vi "Dashboard Main.vi"() -> ()   [LabVIEW 2014]
uses:
  <vilib>/event_ctls.llb/eventvkey.ctl
  <vilib>/Rock Robotics/WPI/Dashboard/WPI_DashboardLogging Global.vi
  <vilib>/Rock Robotics/Network Tables/SD Read Boolean Array.vi
  <vilib>/Rock Robotics/Network Tables/SD Read Number.vi
  <vilib>/Utility/config.llb/Write Key (String).vi
  <vilib>/Utility/config.llb/Write Key (I32).vi
  <vilib>/Utility/config.llb/NI_LVConfig.lvlib
panel:
  in  "TCP":refnum<k5>
  out "Camera IP":string
  out "Image Message":string="Timeout in Camera Communications"
  in  "Dashboard Tab":T1(tab)
  out "Right Joystick Shift":bool
  out "Left Joystick Shift":bool
  out "Right Joystick Arcade":bool
  out "Left Joystick Arcade":bool
  out "Right Joystick X":dbl
  out "Left Joystick Y":dbl
  out "Left Joystick X":dbl
  out "Right Joystick Y":dbl
  out "Intake Open/Close":dbl
  out "Tote Motor Signal":dbl
  out "Tote Elevator Signal":dbl
  out "Top Limit Switch":bool
  out "Bottom Limit Switch":bool
  out "Tote Elevator Pot":dbl
  out "Accelerometer":dbl
  out "Gyro Angle":dbl
  out "Motor Signal":dbl
  out "Encoder":dbl
  out "BR Feedback":dbl
  out "FR Feedback":dbl
  out "BL Feedback":dbl
  out "FL Feedback":dbl
  out "BR Signal":dbl
  out "FR Signal":dbl
  out "BL Signal":dbl
  out "FL Signal":dbl
  in  "Camera Settings":T2={"Frame Rate"=30, "Compression"=30, "Size"=1} {"Frame Rate" scale=1.0..30.0; "Size" items=["640x480", "320x240", "160x120"]}
  out "MotorChart R":cluster{"Numeric":dbl, "Numeric":dbl}(graph)
  out "MotorChart L":T3(graph)
  out "MotorSliders R":cluster{"MotorSlide1":dbl, "MotorSlide2":dbl} {"MotorSlide2" scale=-1.0..1.0 scale format="%#_2e"; "MotorSlide1" scale=-1.0..1.0 scale format="%#_2e"}
  out "MotorSliders L":T4 {"MotorSlide4 2" scale=0.0..14.0 scale format="%#_2e"; "MotorSlide2" scale=-1.0..1.0 scale format="%#_2e"; "MotorSlide1" scale=-1.0..1.0 scale format="%#_2e"}
  out "Gyro":dbl(knob) scale=0.0..360.0
  out "JS1 Z":dbl(slide) scale=-1.0..1.0 scale format="%#_2e"
  out "JS1 Graph":cluster{"X":dbl, "Y":dbl}[](graph)
  out "JS1 Buttons":T5
  out "JS2 Z":dbl(slide) scale=-1.0..1.0 scale format="%#_2e"
  out "JS2 Graph":cluster{"X":dbl, "Y":dbl}[](graph)
  out "JS2 Buttons":T5
  out "Mode":T6(ring)=enum."Auto Disabled"
  in  "DB Camera Config":bool
  out "fps":dbl format="%#.1g"
  out "Mbps":dbl format="%#.1g"
  out "Mbps 2":bool
  out "Camera Image":T7(plugin-control)
  in  "Vision":u16(ring) items=["Camera Off", "USB Camera SW", "USB Camera HW", "IP Camera"]
  in  "Rec Mode":enum32{"Stop", "Record", "Playback"}(radio)
  in  "DB/String 9":string
  in  "DB/String 8":string
  in  "DB/String 7":string
  in  "DB/String 6":string
  in  "DB/String 5":string
  in  "DB/String 4":string
  in  "DB/String 3":string
  in  "DB/String 2":string
  in  "DB/String 1":string
  in  "DB/String 0":string
  in  "DB/Slider 0":dbl(slide) scale=0.0..5.0
  in  "DB/Slider 1":dbl(slide) scale=0.0..5.0
  in  "DB/Slider 2":dbl(slide) scale=0.0..5.0
  in  "DB/Slider 3":dbl(slide) scale=0.0..5.0
  out "DB/LED 3":bool
  out "DB/LED 2":bool
  out "DB/LED 1":bool
  out "DB/LED 0":bool
  in  "DB/Button 3":bool
  in  "DB/Button 2":bool
  in  "DB/Button 1":bool
  in  "DB/Button 0":bool caption="New Name"
  in  "Test Slider":dbl(slide) scale=0.0..100.0 scale format="%#_3g"
  in  "On/Off":bool caption="Solenoid"
  in  "Test Name":u16(ring) items=["Select the test to run...", "Example Test", "-------------------------------", "List of tests is built in robot code.", "Replace with your own automated tests."]
  in  "Test Tree":string(tree)
  in  "Motor":cluster{"Value":dbl, "Enable":bool} {"Value" scale=-1.0..1.0 scale format="%#_3g"}
  out "Progress":T8 {"Test Progress" scale=0.0..100.0}
  in  "Rev/Fwd":cluster{"Forward":bool, "Reverse":bool}
  in  "Test Ring":u16(ring) items=["Monochrome", "Color"]
  in  "Listbox":i32(listbox)
  out "Tree":string(tree)
  out "Boolean":bool
  # "Drivetrain Values"
  # "Other Sensors"
  # "Drivetrain Values"
  # "Craaa"
  # "Tote Elevator"
  # "Tote Intake"
  # "Left"
  # "Front"
  # "Right"
  # "Battery"
  # "This tab is a great place for autonomous settings and robot-specific values.\nPlace controls and indicators inside this tab and match name to\nDashboard Variables on robot. You can also delete this comment."
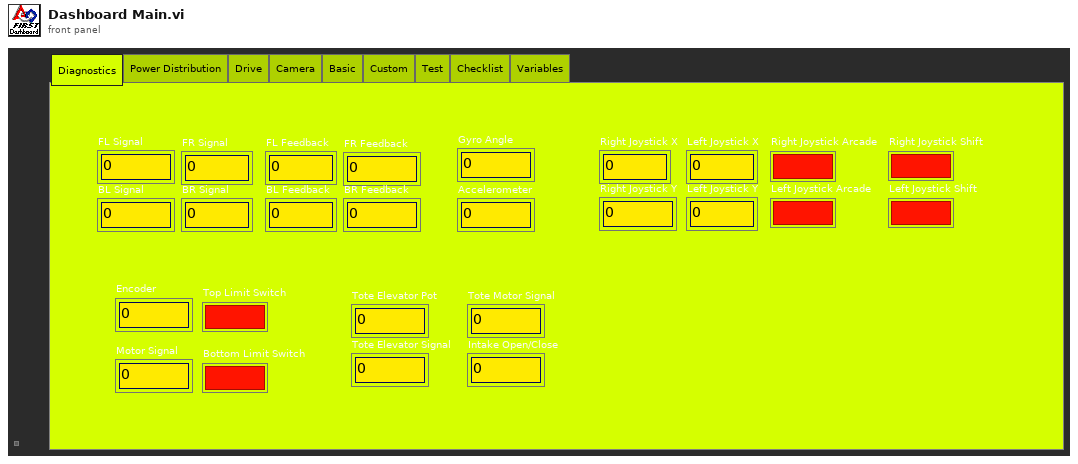
[diagram p1: front panel]
types:
  T1 = enum32{"Diagnostics", "Power Distribution", "Drive", "Camera", "Basic", "Custom", "Test", "Checklist", "Variables"}
  T2 = cluster{"Frame Rate":i32, "Compression":i32, "Size":u16}
  T3 = cluster{"Numeric":dbl, "Numeric":dbl, "Battery V":dbl}
  T4 = cluster{"MotorSlide1":dbl, "MotorSlide2":dbl, "MotorSlide4 2":dbl}
  T5 = cluster{bool, bool, bool, bool, bool, bool, bool, bool, bool, bool, bool, bool}
  T6 = enum8{"Tele-Op Disabled", "Tele-Op Enabled", "Auto Disabled", "Auto Enabled", "Test Disabled", "Test Enabled", "Disconnected", "No Code", "E-Stop"}
  T7 = typedef "IMAQ Image.ctl" = refnum<image>
  T8 = cluster{"Test Progress":u8, "Test Progress Text":string}
  T9 = enum32{"Drive", "Basic", "Custom", "Test", "Checklist", "Variables"}
  T10 = typedef "Image Type" = u32
  T11 = cluster{"Camera Image":refnum<vi>, "Dashboard Tab":refnum<vi>, "Boolean":refnum<vi>, "Vision":refnum<vi>, "Rec Mode":refnum<vi>, "Test Slider":refnum<vi>, "On/Off ":refnum<vi>, "Test Ring":refnum<vi>, "Rev/Fwd":refnum<vi>, "Test Name":refnum<vi>, "Motor":refnum<vi>, "Progress":refnum<vi>, "CheckList":refnum<vi>, "Tree":refnum<vi>, "Test Tree":refnum<vi>}
  T12 = cluster{"Error Strings":string, "Disable Counts":cluster{u16, u16}, "Rail Faults":cluster{u16, u16, u16}, "Robot IP":string, "DB Mode":u8, "Event Info":cluster{"Name":string, "Type":u8, "Number":u16, "Replay":u8}, "Camera Addr":string}
  T13 = cluster{"Storage":cluster{"Disk Free":u64, "RAM Block":u32, "RAM free":u32}, "CPU Utilization":cluster{"CPU % ISR":sgl, "CPU % Time Crit":sgl, "CPU % Timed Str":sgl, "CPU % High":sgl, "CPU % Above":sgl, "CPU % Normal":sgl, "CPU % Low":sgl}, "CAN":cluster{"% Bus Utilization":sgl, "Bus Off Cnt":u32, "TX_FIFO Full Cnt":u32, "Receive Error Cnt":u8, "Transmit Error Cnt":u8}, "HID":cluster{"HID Outputs":u32, "Rumble Low":u16, "Rumble High":u16}[]}
  T14 = cluster{"Status bits":cluster{"Test Mode":bool, "Autonomous":bool, "Enabled":bool, "Code Start":bool, "Brownout":bool, "Reserved 2":bool, "Reserved 3":bool, "E-Stop":bool}, "Code Trace":cluster{"Disabled":bool, "TeleOp":bool, "Auto":bool, "Test":bool}, "Controller Type":enum16{"unknown", "cRIO", "roboRio"}, "Code?":enum16{"unknown", "noCode", "code"}, "Battery V":dbl}
  T15 = cluster{"Control Bits":cluster{"TestMode":bool, "Autonomous":bool, "Enabled":bool, "FMS Present":bool, bool, bool, bool, "E-Stop":bool}, "Team Station ":u8, "Countdown":sgl, "Joystick Values":cluster{"Axes":dbl[], "Buttons":bool[], "POVs":i16[]}[]}
  T16 = cluster{"Axes":dbl[], "Buttons":bool[], "POVs":i16[]}[]
  T17 = cluster{"Axes":dbl[], "Buttons":bool[], "POVs":i16[]}
  T18 = cluster{"Buttons[0]":bool, "Buttons[1]":bool, "Buttons[2]":bool, "Buttons[3]":bool, "Buttons[4]":bool, "Buttons[5]":bool, "Buttons[6]":bool, "Buttons[7]":bool, "Buttons[8]":bool, "Buttons[9]":bool, "Buttons[10]":bool, "Buttons[11]":bool}
  T19 = cluster{"Boolean Array[0]":bool, "Boolean Array[1]":bool, "Boolean Array[2]":bool, "Boolean Array[3]":bool, "Boolean Array[4]":bool, "Boolean Array[5]":bool, "Boolean Array[6]":bool, "Boolean Array[7]":bool, "Boolean Array[8]":bool}
  T20 = cluster{"Numeric Array[0]":dbl, "Numeric Array[1]":dbl, "Numeric Array[2]":dbl, "Numeric Array[3]":dbl, "Numeric Array[4]":dbl, "Numeric Array[5]":dbl, "Numeric Array[6]":dbl, "Numeric Array[7]":dbl, "Numeric Array[8]":dbl}
  T21 = typedef "NI_LVConfig.lvlib/Config Data RefNum.ctl" = refnum<k1>
  T22 = cluster{"Operation":enum16{"Update", "Clear"}, "Color Box":u32}[]
  T23 = typedef "eventvkey.ctl" = enum16{"ASCII", "Enter", "Return", "Shift", "Ctrl", "Alt", "Cmd", "Opt", "Caps", "NumLock", "Clear", "Break", "Up", "Down", "Left", "Right", "Insert", "Delete", "Home", "End", "PageUp", "PageDown", "Escape", "Help", "Pause", "ScrollLock", "F1", "F2", "F3", "F4", "F5", "F6", "F7", "F8", "F9", "F10", "F11", "F12", "F13", "F14", "F15", "F16", "F17", "F18", "F19", "F20", "F21", "F22", "F23", "F24", "Play", "VolumeUp", "VolumeDown", "Mute", "Two Byte Char"}
  T24 = cluster{"Image Size":bool, "Image Type":bool, "Pixel Value":bool, "ROI Information":bool, "Zoom Factor":bool}
  T25 = enum8{"Enabled", "Disabled", "Disabled and Grayed Out"}
  T26 = cluster{"Operation":enum16{"Update", "Clear"}, "Color Box":u32}
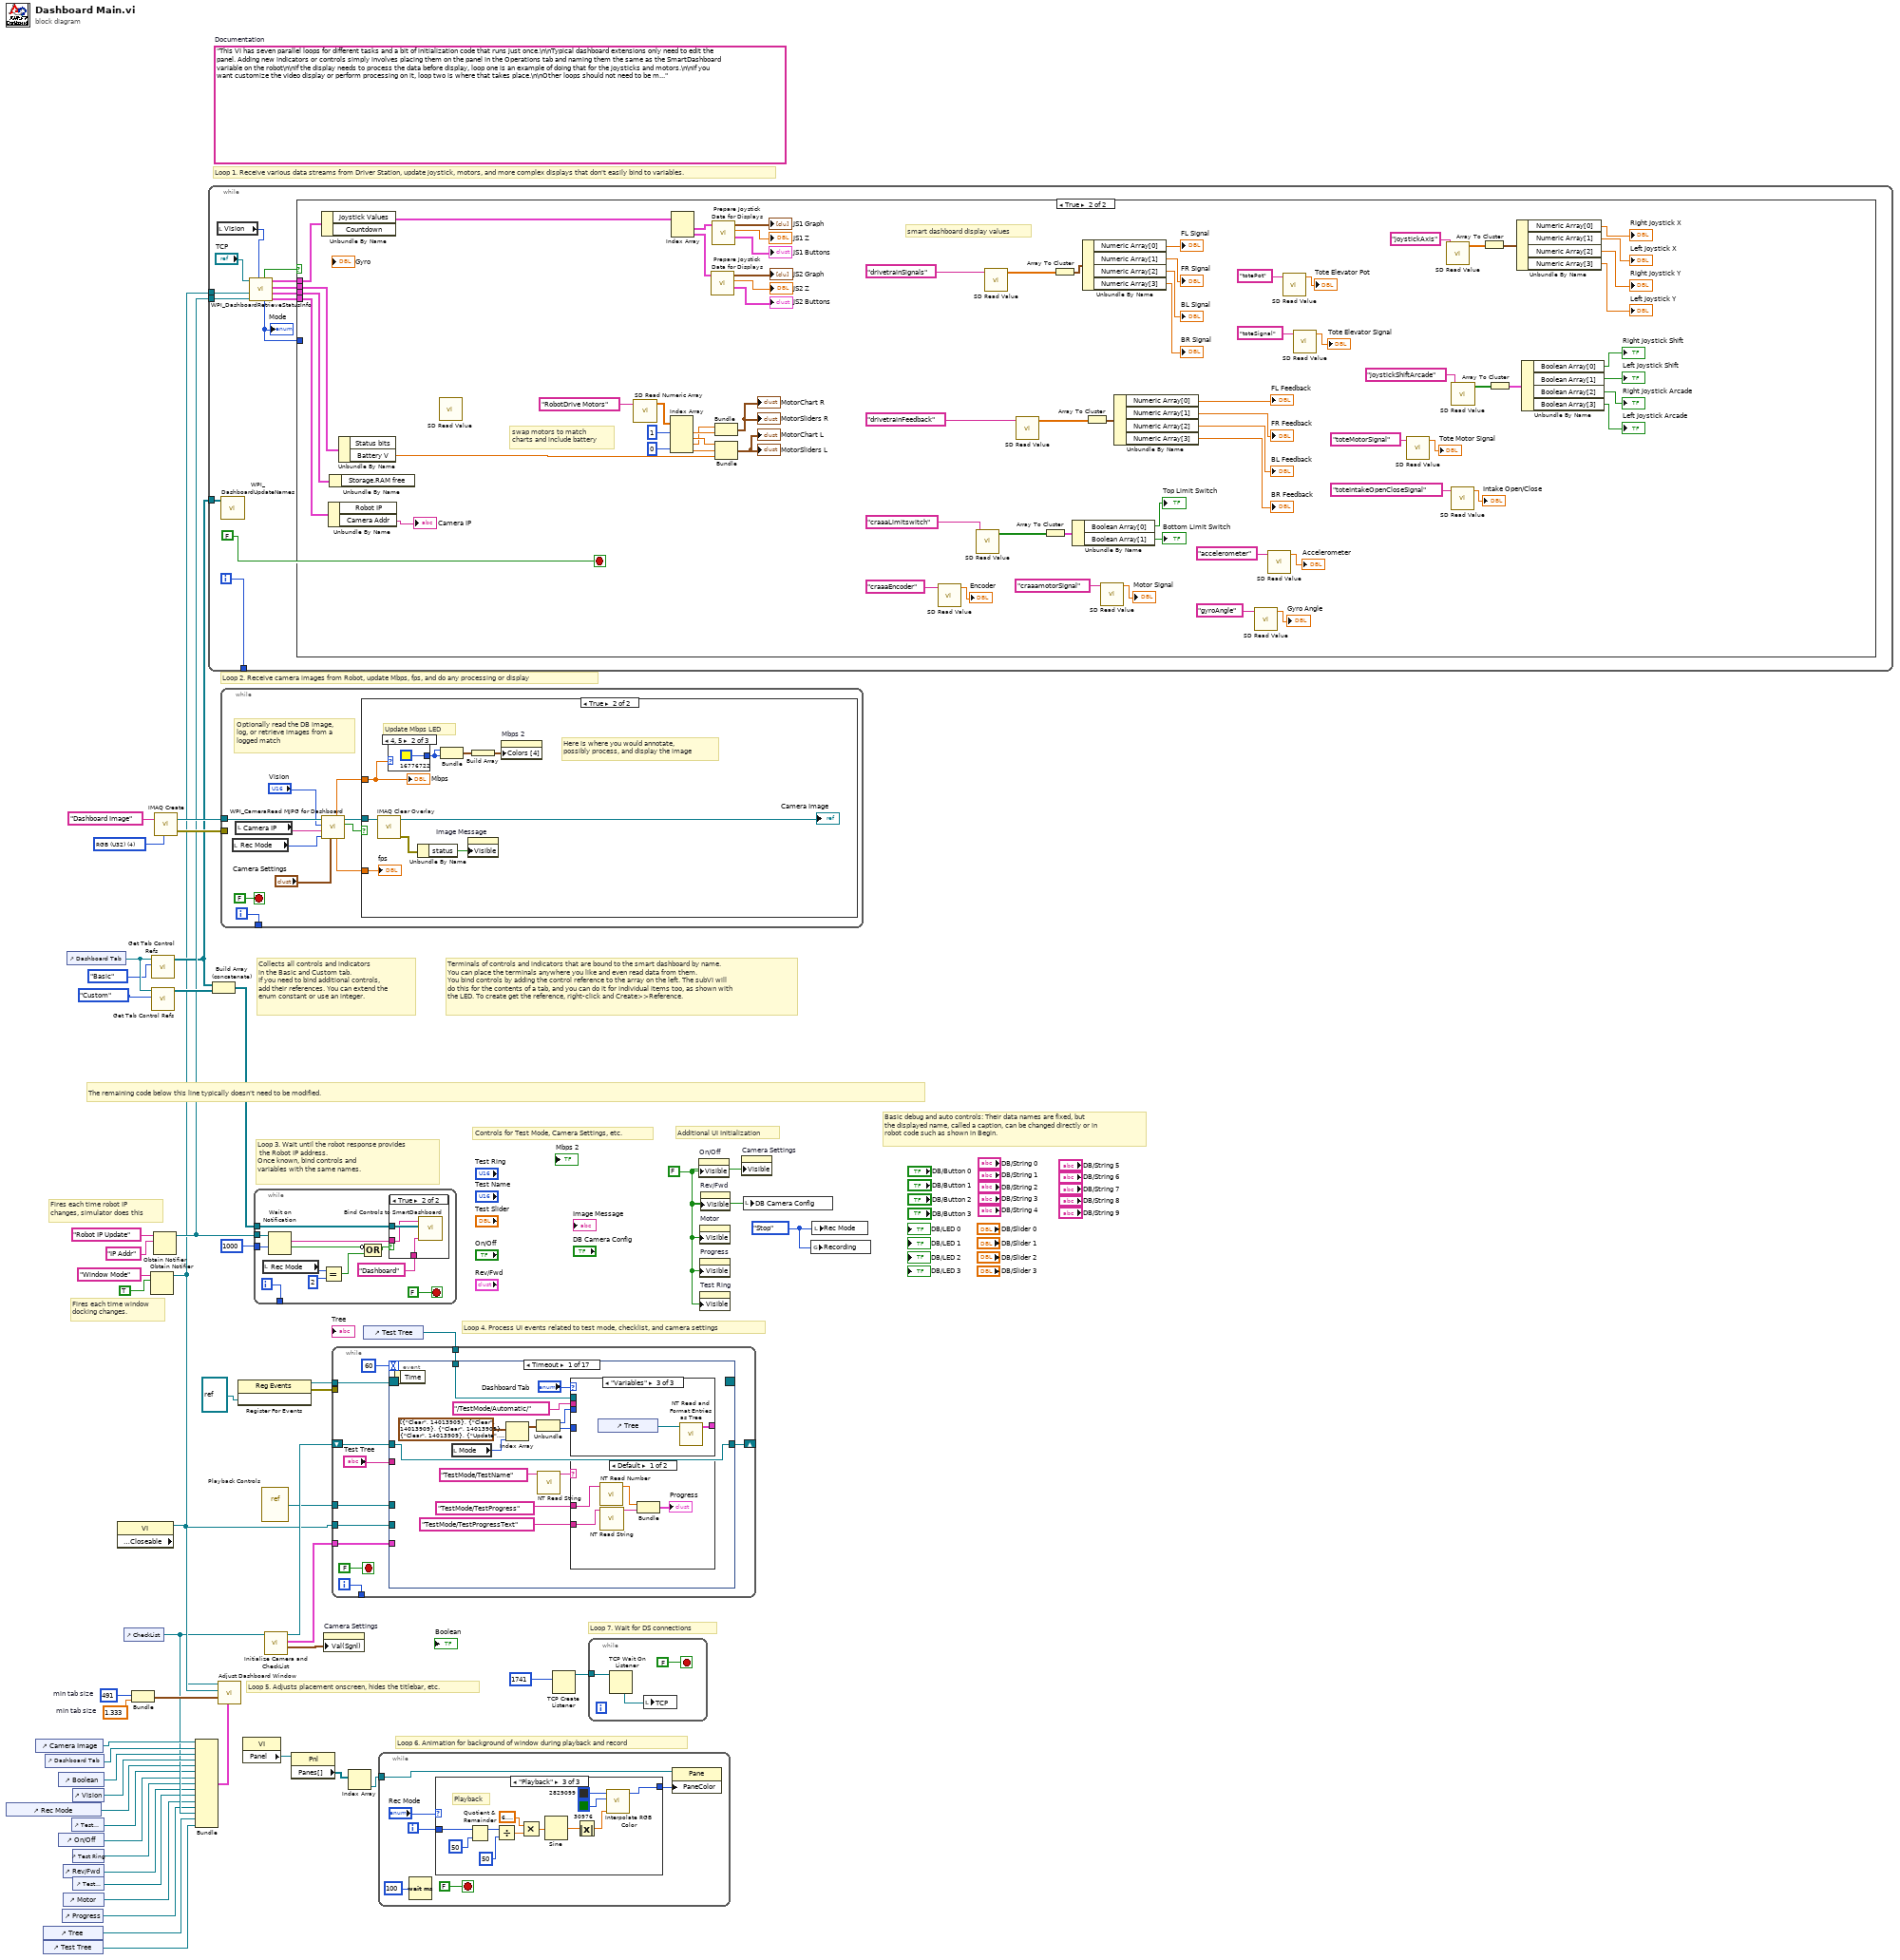
[diagram p0: block diagram]
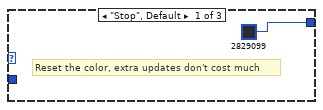
[diagram p3: hidden frame]
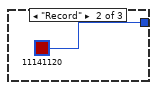
[diagram p4: hidden frame]
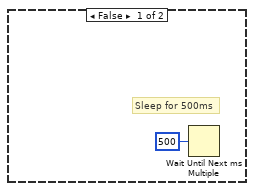
[diagram p6: hidden frame]
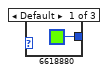
[diagram p7: hidden frame]
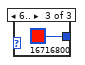
[diagram p8: hidden frame]
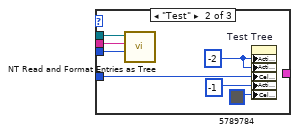
[diagram p10: hidden frame]
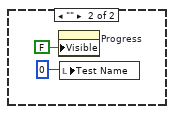
[diagram p11: hidden frame]
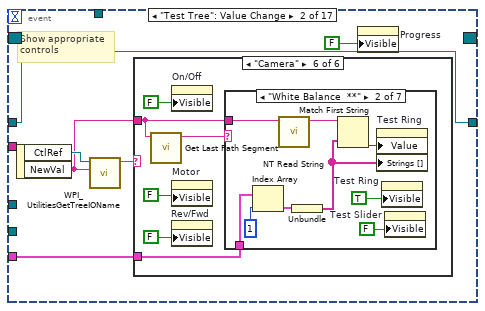
[diagram p12: hidden frame]
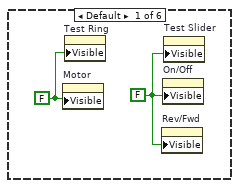
[diagram p13: hidden frame]
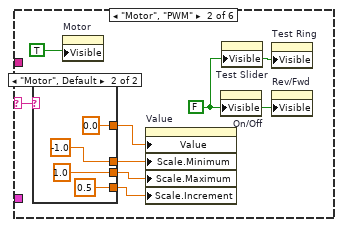
[diagram p14: hidden frame]
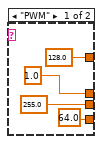
[diagram p15: hidden frame]
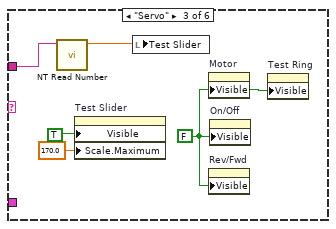
[diagram p16: hidden frame]
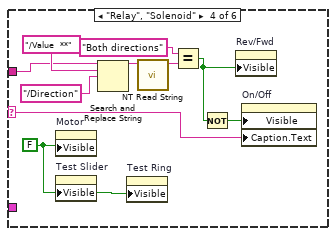
[diagram p17: hidden frame]
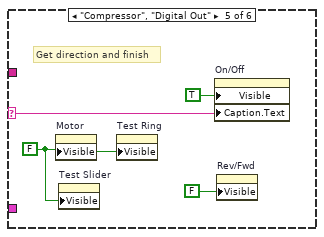
[diagram p18: hidden frame]
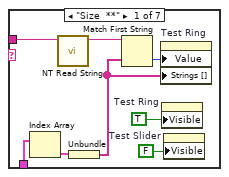
[diagram p19: hidden frame]
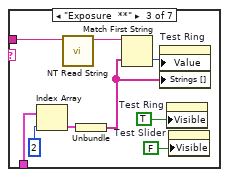
[diagram p20: hidden frame]
diagram:
  w24 = 491  # min tab size
  w23 = 1.333  # min tab size
  w32 = enum32{"Stop", "Record", "Playback"}."Stop" ("Rec Mode")
  w6 = FALSE ("Visible")
  (unwired) "This VI has seven parallel loops for different tasks and a bit of initialization code that runs just once.\n\nTypical dashboard extensions only need to edit the panel. Adding new indicators or controls simply involves placing them on the panel in the Operations tab and naming them the same as the SmartDashboard variable on the robot\n\nIf the display needs to process the data before display, loop one is an example of doing that for the joysticks and motors.\n\nIf you want customize the video display or perform processing on it, loop two is where that takes place.\n\nOther loops should not need to be modified. They are pretty standard, and document the task they perform."  # Documentation
  w52 = T10 4 items=["Grayscale (U8)", "Grayscale (I16)", "Grayscale (SGL)", "Complex (CSG)", "RGB (U32)", "HSL (U32)", "RGB (U64)"] ("Image Type")
  # "Loop 7. Wait for DS connections"
  # "Basic debug and auto controls: Their data names are fixed, but\nthe displayed name, called a caption, can be changed directly or in\nrobot code such as shown in Begin."
  # "Controls for Test Mode, Camera Settings, etc."
  # "Additional UI Initialization"
  # "Loop 6. Animation for background of window during playback and record"
  # "Fires each time robot IP\nchanges, simulator does this"
  # "Fires each time window\ndocking changes."
  # "Collects all controls and indicators\nin the Basic and Custom tab.\nIf you need to bind additional controls,\nadd their references. You can extend the\nenum constant or use an integer."
  # "The remaining code below this line typically doesn't need to be modified."
  # "Loop 4. Process UI events related to test mode, checklist, and camera settings"
  # "Terminals of controls and indicators that are bound to the smart dashboard by name.\nYou can place the terminals anywhere you like and even read data from them.\nYou bind controls by adding the control reference to the array on the left. The subVI will\ndo this for the contents of a tab, and you can do it for individual items too, as shown with\nthe LED. To create get the reference, right-click and Create>>Reference."
  # "Loop 3. Wait until the robot response provides\n the Robot IP address.\nOnce known, bind controls and\nvariables with the same names."
  # "Loop 5. Adjusts placement onscreen, hides the titlebar, etc."
  # "Loop 1. Receive various data streams from Driver Station, update joystick, motors, and more complex displays that don't easily bind to variables."
  # "Loop 2. Receive camera images from Robot, update Mbps, fps, and do any processing or display"
  n1 = control-ref of="Rec Mode"() -> (w12:refnum<vi>)
  n2 = control-ref of="Camera Image"() -> (w27:refnum<vi>)
  n3 = control-ref of="Tree"() -> (w16:refnum<vi>)
  n4 = control-ref of="Test Tree"() -> (w15:refnum<vi>)
  n5 = control-ref of="Dashboard Tab"() -> (w26:refnum<vi>)
  n6 = control-ref of="Boolean"() -> (w21:refnum<vi>)
  n7 = control-ref of="On/Off"() -> (w10:refnum<vi>)
  n8 = control-ref of="Progress"() -> (w7:refnum<vi>)
  n9 = control-ref of="Rev/Fwd"() -> (w8:refnum<vi>)
  n10 = control-ref of="Motor"() -> (w13:refnum<vi>)
  n11 = control-ref of="Dashboard Tab"() -> (w30:refnum<vi>)
  n12 = control-ref of="Test Slider"() -> (w11:refnum<vi>)
  n13 = control-ref of="Vision"() -> (w25:refnum<vi>)
  n14 = control-ref of="Test Ring"() -> (w9:refnum<vi>)
  n15 = control-ref of="Test Name"() -> (w14:refnum<vi>)
  n16 = property class="VI" props=["Front Panel.Closeable"]() -> (reference out=w31:refnum<vi>)  [unwired: 2 in, 2 out]
  n17 = control-ref of="CheckList"() -> (w17:refnum<vi>)
  n18 = Bundle("min tab size"=w24, "min tab size"=w23) -> (w22:cluster{"min tab size":i32, "min tab size":dbl})  [unwired: 1 in]
  n19 = Obtain Notifier(name (unnamed)="Window Mode", notification data type=TRUE) -> (notifier out=w3:refnum<notifier>)  [unwired: 2 in, 2 out]
  n20 = call <vilib>:"Get Tab Control Refs.vi"("Page Index"=T9."Basic" ("Dashboard Tab"), "TabControl in"=w30) -> ("ControlsOnPage"=w4:refnum<vi>[])  [unwired: 9 in]
  n21 = call <vilib>:"Get Tab Control Refs.vi"("Page Index"=T9."Custom" ("Dashboard Tab"), "TabControl in"=w30) -> ("ControlsOnPage"=w29:refnum<vi>[])  [unwired: 9 in]
  n22 = Obtain Notifier(name (unnamed)="Robot IP Update", notification data type="IP Addr" ("name (unnamed)")) -> (notifier out=w5:refnum<notifier>)  [unwired: 2 in, 2 out]
  n23 = call "IMAQ Create"("Image Name"="Dashboard Image", "Image Type"=w52) -> ("New Image"=w50:T7, "error out"=w49:errorcluster)  [unwired: 2 in, 1 out]
  n24 = Bundle("Camera Image"=w27, "Dashboard Tab"=w26, "Boolean"=w21, "Vision"=w25, "Rec Mode"=w12, "Test Slider"=w11, "On/Off"=w10, "Test Ring"=w9, "Rev/Fwd"=w8, "Test Name"=w14, "Motor"=w13, "Progress"=w7, "CheckList"=w17, "Tree"=w16, "Test Tree"=w15) -> (w18:T11)  [unwired: 1 in]
  n25 = while {
    tunnel: [w64] -> _
    tunnel: w5 -> [w58]
    tunnel: w4 -> [w57]
    tunnel: w3 -> [w53]
    i -> [w64]
    stop <- FALSE stop-if-true
    n26 = local read "Vision"() -> (w55:u16)
    n27 = call <vilib>:"WPI_DashboardUpdateNames.vi"("Controls on Tab"=w57) -> ()  [unwired: 11 in]
    n28 = call <vilib>:"WPI_DashboardRetrieveStatusInfo.vi"("Vision"=w55, "Binding Refnum"=w58, "Window Mode Notifier"=w53, "TCP Cnx"="TCP") -> ("Power and Errors"=w59:T12, "Robot Metrics"=w62:T13, "Status Info"=w63:T14, "Control Info"=w60:T15, "Robot Mode"=w56:T6, "Process?"=w61:bool)  [unwired: 2 in]
    "Mode" <- w56
    n29 = case shown="True" w61 {
      tunnel: w63 -> [_ w139]
      tunnel: w62 -> [_ w138]
      tunnel: w60 -> [_ w137]
      tunnel: w59 -> [_ w136]
      tunnel: w56 -> [_ _]
      frame False {
      }
      frame True {
        # "smart dashboard display values"
        # "swap motors to match\ncharts and include battery"
        n30 = Unbundle By Name(w137) -> ("Joystick Values"=w124:T16)  [unwired: 1 out]
        n31 = Unbundle By Name(w136) -> ("Camera Addr"=→"Camera IP":string)  [unwired: 1 out]
        n32 = Unbundle By Name(w138) -> ()  [unwired: 1 out]
        n33 = Unbundle By Name(w139) -> ("Battery V"=w125:dbl)  [unwired: 1 out]
        n34 = call-poly <vilib>:"SD Read Value.vi"() -> ()  [unwired: 9 in, 3 out]
        n35 = call <vilib>:"SD Read Numeric Array.vi"("Name"="RobotDrive Motors") -> ("Numeric Array"=w127:dbl[])  [unwired: 8 in, 2 out]
        n36 = Index Array(array=w127, index #1=1, index #4=0) -> (element #1=w131:dbl, element #2=w132:dbl, element #3=w130:dbl, element #4=w135:dbl)  [unwired: 2 in]
        n37 = Index Array(array=w124) -> (element #1=w123:T17, element #2=w118:T17)  [unwired: 2 in]
        n38 = call "Prepare Joystick Data for Displays.vi"("Joystick Values"=w118) -> ("Buttons"=→"JS2 Buttons":T18, "Z Axis"=→"JS2 Z":dbl, "Cartesian Data"=→"JS2 Graph":cluster{"X axis":dbl, "X axis":dbl}[])  [unwired: 8 in]
        n39 = call "Prepare Joystick Data for Displays.vi"("Joystick Values"=w123) -> ("Buttons"=→"JS1 Buttons":T18, "Z Axis"=→"JS1 Z":dbl, "Cartesian Data"=→"JS1 Graph":cluster{"X axis":dbl, "X axis":dbl}[])  [unwired: 8 in]
        n40 = Bundle("Numeric"=w130, "Numeric"=w131) -> (→"MotorChart R" →"MotorSliders R":cluster{"Numeric":dbl, "Numeric":dbl})  [unwired: 1 in]
        n41 = Bundle("Numeric"=w132, "Numeric"=w135, "Battery V"=w125) -> (→"MotorChart L" →"MotorSliders L":T3)  [unwired: 1 in]
        n42 = call-poly <vilib>:"SD Read Value.vi"("Name"="craaaEncoder") -> ("Numeric"=→"Encoder":dbl)  [unwired: 8 in, 2 out]
        n43 = call-poly <vilib>:"SD Read Value.vi"("Name"="craaaLimitswitch") -> ("Boolean Array"=w100:bool[])  [unwired: 8 in, 2 out]
        n44 = call-poly <vilib>:"SD Read Value.vi"("Name"="drivetrainSignals") -> ("Numeric Array"=w112:dbl[])  [unwired: 8 in, 2 out]
        n45 = call-poly <vilib>:"SD Read Value.vi"("Name"="drivetrainFeedback") -> ("Numeric Array"=w106:dbl[])  [unwired: 8 in, 2 out]
        n46 = Array To Cluster(array=w100) -> (cluster=w99:T19)
        n47 = Array To Cluster(array=w112) -> (cluster=w111:T20)
        n48 = Unbundle By Name(w99) -> ("Boolean Array[0]"=→"Top Limit Switch":bool, "Boolean Array[1]"=→"Bottom Limit Switch":bool)
        n49 = Unbundle By Name(w111) -> ("Numeric Array[0]"=→"FL Signal":dbl, "Numeric Array[1]"=→"FR Signal":dbl, "Numeric Array[2]"=→"BL Signal":dbl, "Numeric Array[3]"=→"BR Signal":dbl)
        n50 = Array To Cluster(array=w106) -> (cluster=w105:T20)
        n51 = call-poly <vilib>:"SD Read Value.vi"("Name"="craaamotorSignal") -> ("Numeric"=→"Motor Signal":dbl)  [unwired: 8 in, 2 out]
        n52 = Unbundle By Name(w105) -> ("Numeric Array[0]"=→"FL Feedback":dbl, "Numeric Array[1]"=→"FR Feedback":dbl, "Numeric Array[2]"=→"BL Feedback":dbl, "Numeric Array[3]"=→"BR Feedback":dbl)
        n53 = call-poly <vilib>:"SD Read Value.vi"("Name"="gyroAngle") -> ("Numeric"=→"Gyro Angle":dbl)  [unwired: 8 in, 2 out]
        n54 = call-poly <vilib>:"SD Read Value.vi"("Name"="accelerometer") -> ("Numeric"=→"Accelerometer":dbl)  [unwired: 8 in, 2 out]
        n55 = call-poly <vilib>:"SD Read Value.vi"("Name"="totePot") -> ("Numeric"=→"Tote Elevator Pot":dbl)  [unwired: 8 in, 2 out]
        n56 = call-poly <vilib>:"SD Read Value.vi"("Name"="toteSignal") -> ("Numeric"=→"Tote Elevator Signal":dbl)  [unwired: 8 in, 2 out]
        n57 = call-poly <vilib>:"SD Read Value.vi"("Name"="toteMotorSignal") -> ("Numeric"=→"Tote Motor Signal":dbl)  [unwired: 8 in, 2 out]
        n58 = call-poly <vilib>:"SD Read Value.vi"("Name"="joystickAxis") -> ("Numeric Array"=w82:dbl[])  [unwired: 8 in, 2 out]
        n59 = call-poly <vilib>:"SD Read Value.vi"("Name"="toteIntakeOpenCloseSignal") -> ("Numeric"=→"Intake Open/Close":dbl)  [unwired: 8 in, 2 out]
        n60 = call-poly <vilib>:"SD Read Value.vi"("Name"="joystickShiftArcade") -> ("Boolean Array"=w74:bool[])  [unwired: 8 in, 2 out]
        n61 = Array To Cluster(array=w82) -> (cluster=w81:T20)
        n62 = Array To Cluster(array=w74) -> (cluster=w75:T19)
        n63 = Unbundle By Name(w81) -> ("Numeric Array[0]"=→"Right Joystick X":dbl, "Numeric Array[1]"=→"Left Joystick X":dbl, "Numeric Array[2]"=→"Right Joystick Y":dbl, "Numeric Array[3]"=→"Left Joystick Y":dbl)
        n64 = Unbundle By Name(w75) -> ("Boolean Array[0]"=→"Right Joystick Shift":bool, "Boolean Array[1]"=→"Left Joystick Shift":bool, "Boolean Array[2]"=→"Right Joystick Arcade":bool, "Boolean Array[3]"=→"Left Joystick Arcade":bool)
      }
    }
  }
  n65 = Build Array (concatenate)(w4, w29) -> (w28:refnum<vi>[])
  n66 = call "Adjust Dashboard Window.vi"("Sizing Refnums"=w18, "Size Constraints"=w22, "VI"=w31, "Notifier in"=w3) -> ()  [unwired: 8 in]
  n67 = while {
    tunnel: w50 -> [w148]
    tunnel: w49 -> [_]
    tunnel: [w149] -> _
    i -> [w149]
    stop <- FALSE stop-if-true
    # "Optionally read the DB image,\nlog, or retrieve images from a\nlogged match"
    n68 = local read "Rec Mode"() -> (w142:enum32{"Stop", "Record", "Playback"})
    n69 = local read "Camera IP"() -> (w140:string)
    n70 = call <vilib>:"WPI_CameraRead MJPG for Dashboard.vi"("Camera Settings"="Camera Settings", "Rec Mode"=w142, "Camera IP"=w140, "Camera Mode"="Vision", "Refnum in"=w148) -> ("Active"=w146:bool, "Refnum out"=w147:T7, "FPS"=w145:dbl, "Bandwidth (Mbps)"=w144:dbl)  [unwired: 3 in]
    n71 = case shown="True" w146 {
      tunnel: w147 -> [_ w155]
      tunnel: w144 -> [_ w154]
      tunnel: w145 -> [_ w152]
      frame False {
        # "Sleep for 500ms"
        n72 = Wait Until Next ms Multiple(millisecond multiple=u32 500) -> ()  [unwired: 1 out]
      }
      frame True {
        # "Here is where you would annotate,\npossibly process, and display the image"
        # "Update Mbps LED"
        n73 = call "IMAQ Clear Overlay"("Image"=w155) -> ("error out"=w159:errorcluster, "Image Out"=→"Camera Image":T7)  [unwired: 2 in, 7 out]
        n74 = case shown="4, 5" w154 {
          tunnel: [u32 6618880 ("Color Box") u32 16776722 ("Color Box") u32 16716800 ("Color Box")] -> w156
          frame Default {
          }
          frame 4, 5 {
          }
          frame 6.. {
          }
        }
        n75 = Unbundle By Name(w159) -> ("status"=w160:bool)
        n76 = Bundle("Color Box"=w156, "Color Box"=w156) -> (w158:cluster{"Color Box":u32, "Color Box":u32})  [unwired: 1 out]
        n77 = property on="Image Message" class="Str"("Visible"=w160) -> ()  [unwired: 2 in, 2 out]
        n78 = Build Array(w158) -> (w157:cluster{"Color Box":u32, "Color Box":u32}[])
        n79 = property on="Mbps 2" class="Bool (strict)"("Colors [4]"=w157) -> ()  [unwired: 2 in, 2 out]
        "Mbps" <- w154
        "fps" <- w152
      }
    }
  }
  n80 = register-events(refnum<vi> refnum) -> (reference out=w36:refnum<event-registration>, error out=w35:errorcluster)  [unwired: 2 in]
  n81 = property class="VI"() -> ("Panel"=w39:refnum<vi>)  [unwired: 2 in, 2 out]
  n82 = while {
    tunnel: w28 -> [w175]
    tunnel: w5 -> [w173]
    tunnel: [w171] -> _
    tunnel: u32 1000 ("milliseconds to wait") -> [w170]
    i -> [w171]
    stop <- FALSE stop-if-true
    n83 = local read "Rec Mode"() -> (w166:enum32{"Stop", "Record", "Playback"})
    n84 = Wait on Notification(notifier=w173, timeout in ms (-1)=w170) -> (notification=w172:string, timed out?=w168:bool)  [unwired: 2 in, 2 out]
    n85 = Equal?(x=w166, y=u16 2 ("Rec Mode")) -> (x = y?=w167:bool)
    n86 = Compound Arithmetic op=OR(invert w168, w167) -> (w169:bool)
    n87 = case shown="True" w169 {
      tunnel: w175 -> [_ w178]
      tunnel: w172 -> [_ w177]
      tunnel: "Dashboard" -> [_ w176]
      frame False {
      }
      frame True {
        n88 = call <vilib>:"Bind Controls to SmartDashboard.vi"("Client Name"=w176, "Bound Control Refs"=w178, "Server IP Address"=w177) -> ()  [unwired: 9 in]
      }
    }
  }
  n89 = vi-ref "Playback Controls.vi"() -> (w37:refnum<vi>)
  n90 = call "Initialize Camera and CheckList.vi"("ListBox in"=w17) -> ("Cluster"=w43:cluster{"value":i32, "value":i32, "index":i32}, "Array"=w44:cluster{string[]}[], "File Refnum"=w42:T21)  [unwired: 8 in]
  n91 = property class="Pnl"(reference=w39) -> ("Panes[]"=w40:refnum<vi>[])  [unwired: 1 in, 2 out]
  n92 = property on="Camera Settings" class="Clust (strict)"("Val(Sgnl)"=w43) -> ()  [unwired: 2 in, 2 out]
  n93 = Index Array(array=w40) -> (element=w38:refnum<vi>)  [unwired: 1 in]
  n94 = control-ref of="Test Tree"() -> (w41:refnum<vi>)
  n95 = while {
    tunnel: w44 -> [w186]
    shift-right: [w185] -> _
    shift-left: w42 -> [w184]
    tunnel: [w183] -> _
    tunnel: w41 -> [w182]
    tunnel: w37 -> [w181]
    tunnel: w36 -> [w180]
    tunnel: w35 -> [_]
    tunnel: w31 -> [w179]
    i -> [w183]
    stop <- FALSE stop-if-true
    n96 = event shown="[0] Timeout" {
      selector: w180 -> [_ _ _ _ _ _ _ _ _ _ _ _ _ _ _ _ _]
      dyn-events: [_ _ _ _ _ _ _ _ _ _ _ _ _ w424 _ _ _] -> _
      timeout: u32 60 ("milliseconds to wait") -> [_ _ _ _ _ _ _ _ _ _ _ _ _ _ _ _ _]
      tunnel: w182 -> [w198 _ _ _ _ _ _ _ _ _ _ _ _ _ _ _ _]
      tunnel: "Test Tree" -> [_ _ _ _ _ _ _ _ w393 w401 w403 w407 w415 _ _ _ _]
      tunnel: w186 -> [_ w220 _ _ _ _ w357 w387 _ _ _ _ _ _ _ _ _]
      tunnel: [w194 w219 w318 w323 w331 w343 w356 w380 w392 w399 w402 w406 w414 w426 w440 w441 w451] -> w185
      tunnel: w184 -> [w194 w219 w318 w323 w331 w343 w355 w380 w392 w399 w402 w406 w414 w426 w440 w441 w451]
      tunnel: w181 -> [_ _ _ _ _ _ _ _ _ _ _ _ _ w427 _ w444 _]
      tunnel: w179 -> [_ _ _ _ _ _ _ _ _ _ _ _ _ w422 _ _ _]
      event Timeout {
        n97 = event-data() -> ()  [unwired: 1 in, 1 out]
        n98 = local read "Mode"() -> (w197:T6)
        n99 = Index Array(array=T22 [{"Operation"=enum."Clear", "Color Box"=14013909}, {"Operation"=enum."Clear", "Color Box"=14013909}, {"Operation"=enum."Clear", "Color Box"=14013909}, {"Operation"=enum."Clear", "Color Box"=14013909}, {"Operation"=enum."Update", "Color Box"=14013909}, {"Operation"=enum."Update", "Color Box"=16777215}, {"Operation"=enum."Clear", "Color Box"=14013909}, {"Operation"=enum."Clear", "Color Box"=14013909}, {"Operation"=enum."Clear", "Color Box"=14013909}], index=w197) -> (element=w192:T26)
        n100 = Unbundle(w192) -> ("Operation"=w191:enum16{"Update", "Clear"}, "Color Box"=w190:u32)
        n101 = call <vilib>:"NT Read String.vi"("Name"="TestMode/TestName") -> ("String"=w201:string)  [unwired: 9 in, 1 out]
        n102 = case shown="\"Variables\"" "Dashboard Tab" {
          tunnel: w198 -> [_ w209 _]
          tunnel: "/TestMode/Automatic/" ("Name Pattern") -> [_ w208 _]
          tunnel: w191 -> [_ w207 _]
          tunnel: [_ _ w211] -> _
          tunnel: w190 -> [_ w203 _]
          frame "Custom", Default {
          }
          frame "Test" {
            w206 = -2 ("Active Item:Row Number")
            n103 = call <vilib>:"NT Read and Format Entries as Tree.vi"("Operation"=w207, "Name Pattern"=w208, "Tree Refnum"=w209) -> ()  [unwired: 7 in, 2 out]
            n104 = property on="Test Tree" class="Tree (strict)"("Active Item Row Number"=w206, "ActiveColNum"=w206, "CellBG"=w203, "Active Item Row Number"=-1 ("Active Item:Row Number"), "CellBG"=u32 5789784 ("Color Box")) -> ()  [unwired: 2 in, 2 out]
          }
          frame "Variables" {
            n105 = control-ref of="Tree"() -> (w210:refnum<vi>)
            n106 = call <vilib>:"NT Read and Format Entries as Tree.vi"("Tree Refnum"=w210) -> ("Formatted Strings"=w211:cluster{"Name":string, "Value":string}[])  [unwired: 9 in, 1 out]
          }
        }
        n107 = case shown="Default" w201 {
          tunnel: "TestMode/TestProgress" ("Name") -> [w213 _]
          tunnel: "TestMode/TestProgressText" ("Name") -> [w212 _]
          frame Default {
            n108 = call <vilib>:"NT Read Number.vi"("Name"=w213) -> ("Numeric"=w214:dbl)  [unwired: 9 in, 1 out]
            n109 = call <vilib>:"NT Read String.vi"("Name"=w212) -> ("String"=w215:string)  [unwired: 9 in, 1 out]
            n110 = Bundle("Numeric"=w214, "String"=w215) -> (→"Progress":cluster{"Numeric":dbl, "String":string})  [unwired: 1 in]
          }
          frame "" {
            n111 = property on="Progress" class="Clust (strict)"("Visible"=FALSE) -> ()  [unwired: 2 in, 2 out]
            n112 = local write "Test Name"(u16 0) -> ()
          }
        }
      }
      event "Test Tree": Value Change {
        # "Show appropriate\ncontrols"
        n113 = event-data() -> ("CtlRef"=w223:refnum<vi>, "NewVal"=w221:string)  [unwired: 1 in]
        n114 = call <vilib>:"WPI_UtilitiesGetTreeIOName.vi"("NewVal"=w221, "TreeControl in"=w223) -> ("I/O Name"=w224:string)  [unwired: 9 in]
        n115 = case shown="\"Camera\"" w224 {
          selector: w224 -> [_ w231 _ w249 w258 _]
          tunnel: w221 -> [_ _ w246 w248 _ w265]
          tunnel: w220 -> [_ _ _ _ _ w264]
          frame Default {
            w226 = FALSE ("Visible")
            w225 = FALSE ("Visible")
            n116 = property on="Motor" class="Clust (strict)"("Visible"=w225) -> ()  [unwired: 2 in, 2 out]
            n117 = property on="Test Ring" class="Ring (strict)"("Visible"=w225) -> ()  [unwired: 2 in, 2 out]
            n118 = property on="Rev/Fwd" class="Clust (strict)"("Visible"=w226) -> ()  [unwired: 2 in, 2 out]
            n119 = property on="On/Off" class="Bool (strict)"("Visible"=w226) -> ()  [unwired: 2 in, 2 out]
            n120 = property on="Test Slider" class="Slide (strict)"("Visible"=w226) -> ()  [unwired: 2 in, 2 out]
          }
          frame "Motor", "PWM" {
            w232 = FALSE ("Visible")
            n121 = case shown="\"Motor\", Default" w231 {
              tunnel: [1.0 ("Value") -1.0 ("Value")] -> w230
              tunnel: [255.0 ("Value") 1.0 ("Value")] -> w229
              tunnel: [128.0 ("Value") 0.0 ("Value")] -> w228
              tunnel: [64.0 ("Value") 0.5 ("Value")] -> w227
              frame "PWM" {
              }
              frame "Motor", Default {
              }
            }
            n122 = property on="Motor" class="Clust (strict)"("Visible"=TRUE) -> ()  [unwired: 2 in, 2 out]
            n123 = property on="Value" class="Slide (strict)"("Value"=w228, "Scale.Minimum"=w230, "Scale.Maximum"=w229, "Scale.Increment"=w227) -> ()  [unwired: 2 in, 2 out]
            n124 = property on="On/Off" class="Bool (strict)"("Visible"=w232) -> ()  [unwired: 2 in, 2 out]
            n125 = property on="Test Slider" class="Slide (strict)"("Visible"=w232) -> ()  [unwired: 2 in, 2 out]
            n126 = property on="Test Ring" class="Ring (strict)"("Visible"=w232) -> ()  [unwired: 2 in, 2 out]
            n127 = property on="Rev/Fwd" class="Clust (strict)"("Visible"=w232) -> ()  [unwired: 2 in, 2 out]
          }
          frame "Servo" {
            w244 = FALSE ("Visible")
            n128 = call <vilib>:"NT Read Number.vi"("Name"=w246) -> ("Numeric"=w245:dbl)  [unwired: 9 in, 1 out]
            n129 = property on="Test Slider" class="Slide (strict)"("Visible"=TRUE, "Scale.Maximum"=170.0 ("Scale.Range:Maximum")) -> ()  [unwired: 2 in, 2 out]
            n130 = local write "Test Slider"(w245) -> ()
            n131 = property on="Motor" class="Clust (strict)"("Visible"=w244) -> ()  [unwired: 2 in, 2 out]
            n132 = property on="Rev/Fwd" class="Clust (strict)"("Visible"=w244) -> ()  [unwired: 2 in, 2 out]
            n133 = property on="On/Off" class="Bool (strict)"("Visible"=w244) -> ()  [unwired: 2 in, 2 out]
            n134 = property on="Test Ring" class="Ring (strict)"("Visible"=w244) -> ()  [unwired: 2 in, 2 out]
          }
          frame "Relay", "Solenoid" {
            w247 = FALSE ("Visible")
            n135 = property on="Motor" class="Clust (strict)"("Visible"=w247) -> ()  [unwired: 2 in, 2 out]
            n136 = property on="Test Slider" class="Slide (strict)"("Visible"=w247) -> ()  [unwired: 2 in, 2 out]
            n137 = Search and Replace String(input string=w248, search string="/Value  **", replace string="/Direction") -> (result string=w254:string)  [unwired: 5 in, 3 out]
            n138 = property on="Test Ring" class="Ring (strict)"("Visible"=w247) -> ()  [unwired: 2 in, 2 out]
            n139 = call <vilib>:"NT Read String.vi"("Name"=w254) -> ("String"=w252:string)  [unwired: 9 in, 1 out]
            n140 = Equal?(x="Both directions", y=w252) -> (x = y?=w250:bool)
            n141 = Not(x=w250) -> (.not. x?=w251:bool)
            n142 = property on="Rev/Fwd" class="Clust (strict)"("Visible"=w250) -> ()  [unwired: 2 in, 2 out]
            n143 = property on="On/Off" class="Bool (strict)"("Visible"=w251, "Caption.Text"=w249) -> ()  [unwired: 2 in, 2 out]
          }
          frame "Compressor", "Digital Out" {
            w257 = FALSE ("Visible")
            # "Get direction and finish"
            n144 = property on="Motor" class="Clust (strict)"("Visible"=w257) -> ()  [unwired: 2 in, 2 out]
            n145 = property on="Test Slider" class="Slide (strict)"("Visible"=w257) -> ()  [unwired: 2 in, 2 out]
            n146 = property on="Test Ring" class="Ring (strict)"("Visible"=w257) -> ()  [unwired: 2 in, 2 out]
            n147 = property on="On/Off" class="Bool (strict)"("Visible"=TRUE, "Caption.Text"=w258) -> ()  [unwired: 2 in, 2 out]
            n148 = property on="Rev/Fwd" class="Clust (strict)"("Visible"=FALSE) -> ()  [unwired: 2 in, 2 out]
          }
          frame "Camera" {
            n149 = call <vilib>:"Get Last Path Segment.vi"("String in"=w265) -> ("String out"=w266:string)  [unwired: 10 in]
            n150 = property on="On/Off" class="Bool (strict)"("Visible"=FALSE) -> ()  [unwired: 2 in, 2 out]
            n151 = property on="Motor" class="Clust (strict)"("Visible"=FALSE) -> ()  [unwired: 2 in, 2 out]
            n152 = property on="Rev/Fwd" class="Clust (strict)"("Visible"=FALSE) -> ()  [unwired: 2 in, 2 out]
            n153 = case shown="\"White Balance  **\"" w266 {
              tunnel: w265 -> [w272 w281 w290 w299 w308 _ w314]
              tunnel: w264 -> [w270 w278 w287 w296 w305 _ _]
              frame "Size  **" {
                n154 = Index Array(array=w270) -> (element=w269:cluster{string[]})  [unwired: 1 in]
                n155 = call <vilib>:"NT Read String.vi"("Name"=w272) -> ("String"=w271:string)  [unwired: 9 in, 1 out]
                n156 = Unbundle(w269) -> (w267:string[])
                n157 = Match First String(2:w267, 3:w271) -> (0:w268:i32)  [unwired: 1 out]
                n158 = property on="Test Ring" class="Ring (strict)"("Value"=w268, "Strings []"=w267) -> ()  [unwired: 2 in, 2 out]
                n159 = property on="Test Ring" class="Ring (strict)"("Visible"=TRUE) -> ()  [unwired: 2 in, 2 out]
                n160 = property on="Test Slider" class="Slide (strict)"("Visible"=FALSE) -> ()  [unwired: 2 in, 2 out]
              }
              frame "White Balance  **" {
                n161 = Index Array(array=w278, index=1) -> (element=w279:cluster{string[]})
                n162 = call <vilib>:"NT Read String.vi"("Name"=w281) -> ("String"=w280:string)  [unwired: 9 in, 1 out]
                n163 = Unbundle(w279) -> (w276:string[])
                n164 = Match First String(2:w276, 3:w280) -> (0:w275:i32)  [unwired: 1 out]
                n165 = property on="Test Ring" class="Ring (strict)"("Value"=w275, "Strings []"=w276) -> ()  [unwired: 2 in, 2 out]
                n166 = property on="Test Ring" class="Ring (strict)"("Visible"=TRUE) -> ()  [unwired: 2 in, 2 out]
                n167 = property on="Test Slider" class="Slide (strict)"("Visible"=FALSE) -> ()  [unwired: 2 in, 2 out]
              }
              frame "Exposure  **" {
                n168 = Index Array(array=w287, index=2) -> (element=w288:cluster{string[]})
                n169 = call <vilib>:"NT Read String.vi"("Name"=w290) -> ("String"=w289:string)  [unwired: 9 in, 1 out]
                n170 = Unbundle(w288) -> (w284:string[])
                n171 = Match First String(2:w284, 3:w289) -> (0:w285:i32)  [unwired: 1 out]
                n172 = property on="Test Ring" class="Ring (strict)"("Value"=w285, "Strings []"=w284) -> ()  [unwired: 2 in, 2 out]
                n173 = property on="Test Ring" class="Ring (strict)"("Visible"=TRUE) -> ()  [unwired: 2 in, 2 out]
                n174 = property on="Test Slider" class="Slide (strict)"("Visible"=FALSE) -> ()  [unwired: 2 in, 2 out]
              }
              frame "Exposure Priority  **" {
                n175 = Index Array(array=w296, index=3) -> (element=w297:cluster{string[]})
                n176 = call <vilib>:"NT Read String.vi"("Name"=w299) -> ("String"=w298:string)  [unwired: 9 in, 1 out]
                n177 = Unbundle(w297) -> (w293:string[])
                n178 = Match First String(2:w293, 3:w298) -> (0:w294:i32)  [unwired: 1 out]
                n179 = property on="Test Ring" class="Ring (strict)"("Value"=w294, "Strings []"=w293) -> ()  [unwired: 2 in, 2 out]
                n180 = property on="Test Ring" class="Ring (strict)"("Visible"=TRUE) -> ()  [unwired: 2 in, 2 out]
                n181 = property on="Test Slider" class="Slide (strict)"("Visible"=FALSE) -> ()  [unwired: 2 in, 2 out]
              }
              frame "Color Enable  **" {
                n182 = Index Array(array=w305, index=4) -> (element=w306:cluster{string[]})
                n183 = call <vilib>:"NT Read String.vi"("Name"=w308) -> ("String"=w307:string)  [unwired: 9 in, 1 out]
                n184 = Unbundle(w306) -> (w302:string[])
                n185 = Match First String(2:w302, 3:w307) -> (0:w303:i32)  [unwired: 1 out]
                n186 = property on="Test Ring" class="Ring (strict)"("Value"=w303, "Strings []"=w302) -> ()  [unwired: 2 in, 2 out]
                n187 = property on="Test Ring" class="Ring (strict)"("Visible"=TRUE) -> ()  [unwired: 2 in, 2 out]
                n188 = property on="Test Slider" class="Slide (strict)"("Visible"=FALSE) -> ()  [unwired: 2 in, 2 out]
              }
              frame Default {
                n189 = property on="Test Ring" class="Ring (strict)"("Visible"=FALSE) -> ()  [unwired: 2 in, 2 out]
                n190 = property on="Test Slider" class="Slide (strict)"("Visible"=FALSE) -> ()  [unwired: 2 in, 2 out]
              }
              frame "Brightness  **", "Color Level  **", "Compression  **", "FPS  **", "Sharpness  **" {
                n191 = call <vilib>:"NT Read Number.vi"("Name"=w314) -> ("Numeric"=w313:dbl)  [unwired: 9 in, 1 out]
                n192 = local write "Test Slider"(w313) -> ()
                n193 = property on="Test Slider" class="Slide (strict)"("Visible"=TRUE, "Scale.Maximum"=100.0 ("Scale.Range:Maximum")) -> ()  [unwired: 2 in, 2 out]
                n194 = property on="Test Ring" class="Ring (strict)"("Visible"=FALSE) -> ()  [unwired: 2 in, 2 out]
              }
            }
          }
        }
        n195 = property on="Progress" class="Clust (strict)"("Visible"=FALSE) -> ()  [unwired: 2 in, 2 out]
      }
      event "Test Name": Mouse Enter {
        # "Populate the ring with the list of tests"
        n196 = event-data() -> ()  [unwired: 1 in, 1 out]
        n197 = call <vilib>:"NT Read String Array.vi"("Name"="TestMode/TestList") -> ("String Array"=w322:string[])  [unwired: 9 in, 1 out]
        n198 = Build Array (concatenate)("Select the test to run...", w322) -> (w321:string[])
        n199 = property on="Test Name" class="Ring (strict)"("Strings []"=w321) -> ()  [unwired: 2 in, 2 out]
      }
      event "Test Name": Value Change {
        w324 = FALSE ("Visible")
        # "Tell the robot the test name to run"
        n200 = event-data() -> ("NewVal"=w328:u16)  [unwired: 1 in]
        n201 = property on="Test Name" class="Ring (strict)"() -> ("Strings []"=w329:string[])  [unwired: 2 in, 2 out]
        n202 = local write "Progress"(T8 {"Test Progress"=0, "Test Progress Text"=""} ("Progress")) -> ()
        n203 = Index Array(array=w329, index=w328) -> (element=w327:string)
        n204 = call <vilib>:"NT Write String.vi"("String"=w327, "Name"="TestMode/TestName") -> ()  [unwired: 9 in, 1 out]
        n205 = property on="Progress" class="Clust (strict)"("Visible"=TRUE) -> ()  [unwired: 2 in, 2 out]
        n206 = property on="Motor" class="Clust (strict)"("Visible"=w324) -> ()  [unwired: 2 in, 2 out]
        n207 = property on="Test Slider" class="Slide (strict)"("Visible"=w324) -> ()  [unwired: 2 in, 2 out]
        n208 = property on="On/Off" class="Bool (strict)"("Visible"=w324) -> ()  [unwired: 2 in, 2 out]
        n209 = property on="Rev/Fwd" class="Clust (strict)"("Visible"=w324) -> ()  [unwired: 2 in, 2 out]
        n210 = property on="Test Ring" class="Ring (strict)"("Visible"=w324) -> ()  [unwired: 2 in, 2 out]
      }
      event "Listbox": Double Click {
        # "Shift clears all"
        # "Update symbols on the listbox"
        n211 = event-data() -> ("PlatMods.Shift"=w332:bool, "Row"=w334:i32)  [unwired: 1 in]
        n212 = case shown="True" w332 {
          tunnel: w334 -> [w338 _]
          tunnel: 1 -> [w337 _]
          frame False {
            n213 = property on="Listbox" class="LstBox (strict)"() -> ("Item Symbols"=w336:i32[])  [unwired: 2 in, 2 out]
            n214 = Replace Array Subset(array=w336, new element=w337, index=w338) -> (w335:i32[])
            n215 = property on="Listbox" class="LstBox (strict)"("Item Symbols"=w335) -> ()  [unwired: 2 in, 2 out]
          }
          frame True {
            w339 = 0 ("Top Row")
            n216 = property on="Listbox" class="LstBox (strict)"() -> ("Number of Rows"=w341:u32)  [unwired: 2 in, 2 out]
            n217 = Initialize Array(0, w341) -> (w340:i32[])
            n218 = property on="Listbox" class="LstBox (strict)"("Top Row"=w339, "Value"=w339, "Item Symbols"=w340) -> ()  [unwired: 2 in, 2 out]
          }
        }
      }
      event "Listbox": Key Down {
        # "Update symbols on the listbox\nLeft and right keys check and uncheck"
        n219 = event-data() -> ("VKey"=w345:T23)  [unwired: 1 in]
        n220 = case shown="\"Left\", \"Right\"" w345 {
          selector: w345 -> [w350 _]
          tunnel: eventvkey."Left" ("VKey") -> [w348 _]
          frame "Left", "Right" {
            n221 = Equal?(x=w348, y=w350) -> (x = y?=w349:bool)
            n222 = Select(t=0, s=w349, f=1) -> (s? t:f=w351:i32)
            n223 = property on="Listbox" class="LstBox (strict)"() -> ("Item Symbols"=w354:i32[])  [unwired: 2 in, 2 out]
            n224 = Replace Array Subset(array=w354, new element=w351, index="Listbox") -> (w353:i32[])
            n225 = property on="Listbox" class="LstBox (strict)"("Item Symbols"=w353) -> ()  [unwired: 2 in, 2 out]
          }
          frame Default {
          }
        }
      }
      event "DB Camera Config": Value Change {
        # "Show or hide the cluster of controls, store in ini file"
        n226 = event-data() -> ("NewVal"=w358:bool)  [unwired: 1 in]
        n227 = case shown="False" w358 {
          tunnel: w357 -> [w367 _]
          tunnel: [w360 w378] -> w356
          tunnel: w355 -> [w359 w378]
          frame False {
            w374 = "Camera"
            w377 = FALSE ("Visible")
            n228 = local read "Camera Settings"() -> (w366:T2)
            n229 = Index Array(array=w367) -> (element=w370:cluster{string[]})  [unwired: 1 in]
            n230 = Unbundle(w366) -> ("Frame Rate"=w365:i32, "Compression"=w364:i32, "Size"=w368:u16)
            n231 = Unbundle(w370) -> (w369:string[])
            n232 = Index Array(array=w369, index=w368) -> (element=w363:string)
            n233 = call-poly <vilib>:"Write Key.vi"("section"=w374, "value"=w363, "key"="Size", "refnum"=w359) -> ("refnum out"=w376:T21)  [unwired: 2 in, 5 out]
            n234 = call-poly <vilib>:"Write Key.vi"("section"=w374, "value"=w365, "key"="FrameRate", "refnum"=w376) -> ("refnum out"=w375:T21)  [unwired: 1 in, 6 out]
            n235 = property on="Camera Settings" class="Clust (strict)"("Visible"=w377) -> ()  [unwired: 2 in, 2 out]
            n236 = local write "DB Camera Config"(w377) -> ()
            n237 = call-poly <vilib>:"Write Key.vi"("section"=w374, "value"=w364, "key"="Compression", "refnum"=w375) -> ("refnum out"=w361:T21)  [unwired: 1 in, 6 out]
            n238 = call <vilib>:"Close Config Data.vi"("refnum"=w361) -> ("file path"=w362:path)  [unwired: 2 in, 8 out]
            n239 = call <vilib>:"Open Config Data.vi"("configuration file path"=w362) -> ("refnum"=w360:T21)  [unwired: 8 in, 2 out]
          }
          frame True {
            n240 = property on="Camera Settings" class="Clust (strict)"("Visible"=TRUE) -> ()  [unwired: 2 in, 2 out]
          }
        }
      }
      event "Camera Settings": Value Change {
        # "Update summary string when any elements of DB camera change"
        n241 = event-data() -> ("NewVal"=w391:T2)  [unwired: 1 in]
        n242 = Index Array(array=w387) -> (element=w386:cluster{string[]})  [unwired: 1 in]
        n243 = Unbundle(w391) -> ("Frame Rate"=w382:i32, "Compression"=w381:i32, "Size"=w384:u16)
        n244 = Unbundle(w386) -> (w385:string[])
        n245 = Index Array(array=w385, index=w384) -> (element=w383:string)
        n246 = Format Into String(format string="%s   %dfps   %d%%", w383, w382, w381) -> (resulting string=w388:string)  [unwired: 2 in, 1 out]
        n247 = Build Array(w388) -> (w389:string[])
        n248 = property on="DB Camera Config" class="Bool (strict)"("Strings [4]"=w389) -> ()  [unwired: 2 in, 2 out]
      }
      event "Motor.Enable": Value Change {
        # "When the test mode otor enable helper is set, update that\ntree row item's value"
        n249 = event-data() -> ("NewVal"=w397:bool)  [unwired: 1 in]
        n250 = Unbundle("Motor") -> ("Value"=w396:dbl)  [unwired: 1 out]
        n251 = Select(t=w396, s=w397, f=0.0) -> (s? t:f=w394:dbl)
        n252 = call <vilib>:"NT Write Number.vi"("Numeric"=w394, "Name"=w393) -> ()  [unwired: 9 in, 1 out]
      }
      event "Test Slider": Value Change {
        # "When the test mode slider helper is set, update that\ntree row item's value"
        n253 = event-data() -> ("NewVal"=w400:dbl)  [unwired: 1 in]
        n254 = call <vilib>:"NT Write Number.vi"("Numeric"=w400, "Name"=w401) -> ()  [unwired: 9 in, 1 out]
      }
      event "On/Off": Value Change {
        # "When the test mode on/off helper value is set, update that\ntree row item's value"
        n255 = event-data() -> ("NewVal"=w405:bool)  [unwired: 1 in]
        n256 = Boolean To (0,1)(Boolean=w405) -> (0, 1=w404:i16)
        n257 = call <vilib>:"NT Write Number.vi"("Numeric"=w404, "Name"=w403) -> ()  [unwired: 9 in, 1 out]
      }
      event "Rev/Fwd": Value Change {
        # "When the test mode helper value for relays is set, update that\ntree row item's value"
        n258 = event-data() -> ("NewVal.Forward"=w413:bool, "NewVal.Reverse"=w412:bool)  [unwired: 1 in]
        n259 = Boolean To (0,1)(Boolean=w413) -> (0, 1=w409:i16)
        n260 = Boolean To (0,1)(Boolean=w412) -> (0, 1=w411:i16)
        n261 = Negate(x=w411) -> (-x=w410:i16)
        n262 = Add(x=w409, y=w410) -> (x+y=w408:i16)
        n263 = call <vilib>:"NT Write Number.vi"("Numeric"=w408, "Name"=w407) -> ()  [unwired: 9 in, 1 out]
      }
      event "Test Ring": Value Change {
        # "When a test mode helper value is selected from the ring,\nset the tree item's variable to the string value"
        n264 = event-data() -> ("NewVal"=w417:u16)  [unwired: 1 in]
        n265 = property on="Test Ring" class="Ring (strict)"() -> ("Strings []"=w418:string[])  [unwired: 2 in, 2 out]
        n266 = Index Array(array=w418, index=w417) -> (element=w416:string)
        n267 = call <vilib>:"NT Write String.vi"("String"=w416, "Name"=w415) -> ()  [unwired: 9 in, 1 out]
      }
      event "Rec Mode": Value Change {
        # "Update globals for recording mode and path to read log from.\nClear when logging and let NetworkTables set path for vision to\nuse."
        n268 = event-data() -> ("NewVal"=w428:enum32{"Stop", "Record", "Playback"})  [unwired: 1 in]
        n269 = global write "WPI_DashboardLogging Global.vi" "Logging Filename"(path "") -> ()
        n270 = case shown="\"Playback\"" w428 {
          tunnel: w427 -> [_ w430 w438]
          tunnel: [_ _ w437] -> w424
          tunnel: [_ _ w436] -> _
          tunnel: w422 -> [_ _ w434]
          tunnel: cluster{i32, i32} {-250, 170} -> [_ _ w433]
          tunnel: [_ _ T24 {"Image Size"=TRUE, "Image Type"=TRUE, "Pixel Value"=TRUE, "ROI Information"=TRUE, "Zoom Factor"=FALSE} ("Image Information Shown:All Elements")] -> w420
          tunnel: [_ _ TRUE ("Zoom Factor")] -> w419
          frame Default {
          }
          frame "Stop", "Record" {
            # "Place Window too"
            n271 = invoke class="VI" method="FP.Close"(reference=w430) -> (reference out=w429:refnum<vi>)  [unwired: 2 in, 2 out]
            n272 = invoke class="VI" method="Abort VI"(reference=w429) -> ()  [unwired: 2 in, 3 out]
          }
          frame "Playback" {
            n273 = call "Open Playback Panel.vi"("Offset"=w433, "DB VI Ref"=w434, "Playback in"=w438) -> ("Playback out"=w435:refnum<vi>)  [unwired: 8 in]
            n274 = register-events(w435) -> (reference out=w437:refnum<event-registration>, error out=w436:errorcluster)  [unwired: 2 in]
          }
        }
        n275 = global write "WPI_DashboardLogging Global.vi" "Recording"(w428) -> ()
        n276 = property on="Camera Image" class="ImageControl"("Image Information Shown"=w420, "Image Information Visible"=w419) -> ()  [unwired: 2 in, 2 out]
        n277 = call <vilib>:"WPI_DashboardNT Log FieldName Cache.vi"("Operation"=enum16{"Lookup/Add", "Index", "Clear"}."Clear") -> ()  [unwired: 8 in, 3 out]
      }
      event Panel Close {
        w439 = enum32{"Stop", "Record", "Playback"}."Stop" ("Rec Mode")
        # "Playback window has been closed, abort"
        n278 = event-data() -> ()  [unwired: 1 in, 4 out]
        n279 = local write "Rec Mode"(w439) -> ()
        n280 = global write "WPI_DashboardLogging Global.vi" "Recording"(w439) -> ()
      }
      event Panel Close {
        # "Abort playback window and ourself"
        n281 = event-data() -> ()  [unwired: 1 in, 4 out]
        n282 = invoke class="VI" method="FP.Close"(reference=w444) -> (reference out=w443:refnum<vi>)  [unwired: 2 in, 2 out]
        n283 = invoke class="VI" method="Abort VI"(reference=w443) -> (error out=w442:errorcluster)  [unwired: 2 in, 2 out]
        n284 = invoke class="VI" method="Abort VI"(error in=w442) -> ()  [unwired: 2 in, 3 out]
      }
      event "Vision": Value Change {
        # "Enable/Disable Compression slider.\nHW USB is hard-coded into the camera"
        n285 = event-data() -> ("NewVal"=w450:u16)  [unwired: 1 in]
        n286 = Equal?(x=w450, y=u32 2 ("milliseconds to wait")) -> (x = y?=w448:bool)
        n287 = Select(t=T25."Disabled and Grayed Out" ("Disabled"), s=w448, f=T25."Enabled" ("Disabled")) -> (s? t:f=w445:T25)
        n288 = property on="Compression" class="Slide (strict)"("DisabledEnum"=w445) -> ()  [unwired: 2 in, 2 out]
      }
    }
  }
  n289 = while {
    tunnel: w38 -> [w453]
    i -> [w456]
    stop <- FALSE stop-if-true
    n290 = Wait (ms)(milliseconds to wait=u32 100) -> ()  [unwired: 1 out]
    n291 = case shown="\"Playback\"" "Rec Mode" {
      tunnel: w456 -> [_ _ w471]
      tunnel: [u32 2829099 ("Base Color") u32 11141120 ("Target Color") w460] -> w452
      frame "Stop", Default {
        # "Reset the color, extra updates don't cost much"
      }
      frame "Record" {
      }
      frame "Playback" {
        # "Playback"
        n292 = Quotient & Remainder(x=w471, y=u32 50 ("milliseconds to wait")) -> (x-y*floor(x/y)=w467:u32)  [unwired: 1 out]
        n293 = Divide(x=w467, y=u32 50 ("milliseconds to wait")) -> (x/y=w464:dbl)
        n294 = Multiply(x=6.283185307179586, y=w464) -> (x*y=w469:dbl)
        n295 = Sine(x=w469) -> (sin(x)=w468:dbl)
        n296 = Absolute Value(x=w468) -> (abs(x)=w461:dbl)
        n297 = call "Interpolate RGB Color.vi"("Proportion"=w461, "Target Color"=u32 30976, "Base Color"=u32 2829099) -> ("Result Color"=w460:u32)  [unwired: 8 in]
      }
    }
    n298 = property class="Pane"(reference=w453, "PaneColor"=w452) -> ()  [unwired: 1 in, 2 out]
  }
  n299 = TCP Create Listener(10:u16 1741 ("timeout ms (25000)")) -> (3:w1:refnum<k5>)  [unwired: 4 in, 2 out]
  n300 = while {
    tunnel: w1 -> [w473]
    stop <- FALSE stop-if-true
    n301 = TCP Wait On Listener(11:w473) -> (4:w472:refnum<k5>)  [unwired: 3 in, 4 out]
    n302 = local write "TCP"(w472) -> ()
  }
  n303 = property on="On/Off" class="Bool (strict)"("Visible"=w6) -> ()  [unwired: 2 in, 2 out]
  n304 = property on="Motor" class="Clust (strict)"("Visible"=w6) -> ()  [unwired: 2 in, 2 out]
  n305 = property on="Progress" class="Clust (strict)"("Visible"=w6) -> ()  [unwired: 2 in, 2 out]
  n306 = property on="Test Ring" class="Ring (strict)"("Visible"=w6) -> ()  [unwired: 2 in, 2 out]
  n307 = property on="Rev/Fwd" class="Clust (strict)"("Visible"=w6) -> ()  [unwired: 2 in, 2 out]
  n308 = property on="Camera Settings" class="Clust (strict)"("Visible"=w6) -> ()  [unwired: 2 in, 2 out]
  n309 = local write "DB Camera Config"(w6) -> ()
  n310 = global write "WPI_DashboardLogging Global.vi" "Recording"(w32) -> ()
  n311 = local write "Rec Mode"(w32) -> ()
